vi "nextTrack.vi"(8 "error in (no error)":errorcluster, 11 "Player in":refnum<class "Player.lvclass">) -> (0 "error out":errorcluster, 2 "Song":string, 3 "Player out":refnum<class "Player.lvclass">)   [LabVIEW 2017, in "Player.lvclass"]
uses:
  Player.lvclass
  Player.lvclass/Player.ctl
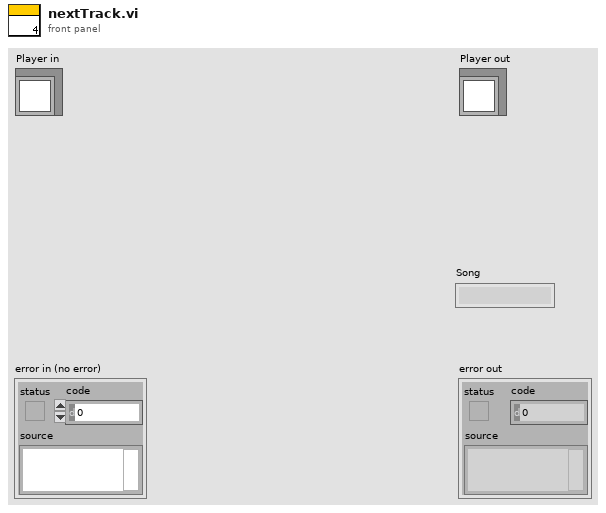
[diagram p1: front panel]
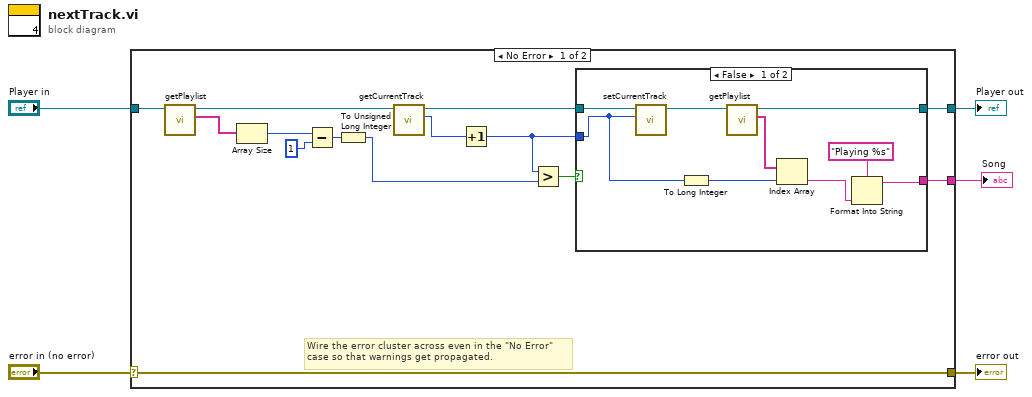
[diagram p0: block diagram]
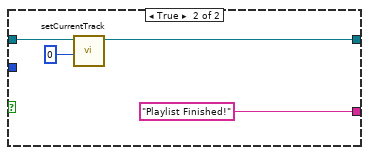
[diagram p2: hidden frame]
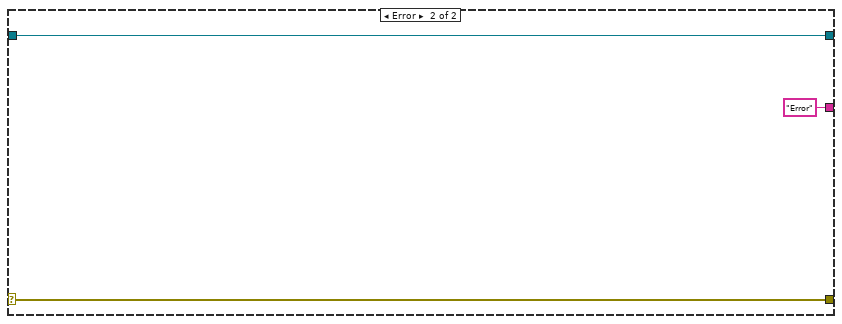
[diagram p3: hidden frame]
diagram:
  n1 = case shown="No Error" "error in (no error)" {
    selector: "error in (no error)" -> [w18 w35]
    tunnel: [w18 w35] -> w4
    tunnel: [w12 w34] -> w2
    tunnel: "Player in" -> [w19 w34]
    tunnel: [w10 "Error"] -> w1
    frame No Error {
      # "Wire the error cluster across even in the \"No Error\"\ncase so that warnings get propagated."
      n2 = call "getPlaylist.vi"("Player in"=w19) -> ("Playlist"=w16:string[], "Player out"=w17:refnum<class "Player.lvclass">)  [unwired: 8 in, 1 out]
      n3 = Array Size(array=w16) -> (size(s)=w15:i32)
      n4 = Subtract(x=w15, y=1) -> (x-y=w13:i32)
      n5 = To Unsigned Long Integer(number=w13) -> (unsigned 32bit integer=w8:u32)
      n6 = call "getCurrentTrack.vi"("Player in"=w17) -> ("currentTrack"=w7:u32, "Player out"=w9:refnum<class "Player.lvclass">)  [unwired: 8 in, 1 out]
      n7 = Increment(x=w7) -> (x+1=w6:u32)
      n8 = Greater?(x=w6, y=w8) -> (0:w11:bool)
      n9 = case shown="False" w11 {
        tunnel: w9 -> [w28 w32]
        tunnel: [w26 w31] -> w12
        tunnel: [w22 "Playlist Finished!"] -> w10
        tunnel: w6 -> [w24 _]
        frame False {
          n10 = call "setCurrentTrack.vi"("currentTrack"=w24, "Player in"=w28) -> ("Player out"=w27:refnum<class "Player.lvclass">)  [unwired: 8 in, 1 out]
          n11 = To Long Integer(number=w24) -> (32bit integer=w23:i32)
          n12 = call "getPlaylist.vi"("Player in"=w27) -> ("Playlist"=w25:string[], "Player out"=w26:refnum<class "Player.lvclass">)  [unwired: 8 in, 1 out]
          n13 = Index Array(array=w25, index=w23) -> (element=w21:string)
          n14 = Format Into String(format string="Playing %s", w21) -> (resulting string=w22:string)  [unwired: 2 in, 1 out]
        }
        frame True {
          n15 = call "setCurrentTrack.vi"("currentTrack"=u32 0, "Player in"=w32) -> ("Player out"=w31:refnum<class "Player.lvclass">)  [unwired: 8 in, 1 out]
        }
      }
    }
    frame Error {
    }
  }
  "error out" <- w4
  "Player out" <- w2
  "Song" <- w1
